vi "ArmSim.vi"(11 "Motor Dmd":dbl) -> (1 "Velocity_RadsPerSec":dbl, 2 "ArmAngle_Rad":dbl)   [LabVIEW 2023]
uses:
  <vilib>/Rock Robotics/WPI/ThirdParty/JAS_Junk/TrajLib/Enum/DCMOTOR_TYPES_ENUM.ctl
  <vilib>/Rock Robotics/WPI/ThirdParty/JAS_Junk/TrajLib/BatterySim_CalculateLoadedBatteryVoltage.vi
  <vilib>/Rock Robotics/WPI/ThirdParty/JAS_Junk/TrajLib/Trajectory_Library.lvlib
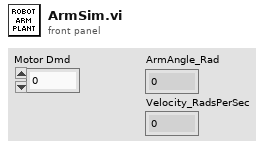
[diagram p1: front panel]
types:
  T1 = typedef "Trajectory_Library.lvlib/DCMOTOR_TYPES_ENUM.ctl" = enum16{"CIM", "AndyMark 9015", "Andy Mark RS 775 125", "Bag", "BaneBots RS 550", "BaneBots RS 775", "Falcon 500", "Mini CIM", "NEO", "NEO 550", "Romi BuiltIn", "Vex 775 Pro", "Snow Blower AM 2235A", "Bosch Seat AM 3493"}
  T2 = typedef "Trajectory_Library.lvlib/SINGLE_JOINT_ARM_SIM_SIMULATION_PARAMS.ctl" = cluster{"MinAngle_Rad":dbl, "MaxAngle_Rad":dbl, "Measurment StdDev":dbl, "SimulateGravity":bool}
  T3 = typedef "Trajectory_Library.lvlib/LINEAR_SYSTEM_ID_SINGLE_JOINT_ARM_MODEL.ctl" = cluster{"DCMOTOR_TYPES":T1, "Num Motors":i32, "ArmLength_M":dbl, "massKg":dbl, "Gearing":dbl, "MOI kgm2":dbl, "Estimate MOI":bool}
  T4 = typedef "Trajectory_Library.lvlib/SINGLE_JOINT_ARM_SIM.ctl" = cluster{"Arm_LinearSystem":T5, "GearBox":T8, "Gearing":dbl, "R_ArmLength_M":dbl, "MinAngle_Rad":dbl, "MaxAngle_Rad":dbl, "SimulateGravity":bool}
  T5 = typedef "Trajectory_Library.lvlib/LINEAR_SYSTEM_SIM.ctl" = cluster{"m_Plant":T6, "m_X":T7, "m_Y":T7, "m_U":T7, "MeasureStdDev":T7}
  T6 = typedef "Trajectory_Library.lvlib/LINEAR_SYSTEM.ctl" = cluster{"m_A":T7, "m_B":T7, "m_C":T7, "m_D":T7, "States":i32, "Inputs":i32, "Outputs":i32}
  T7 = typedef "NI_Matrix.lvlib/RealMatrix.ctl" = dbl[][]
  T8 = typedef "Trajectory_Library.lvlib/DCMOTOR.CTL" = cluster{"nominalVoltage_Volts":dbl, "StallTorque_NM":dbl, "StallCurrent_Amps":dbl, "FreeCurrent_Amps":dbl, "FreeSpeed_RadPerSec":dbl, "R_Ohms":dbl, "KvINV_RadPerSecPerVolt":dbl, "Kt_NMPerAmp":dbl, "L_H":dbl, "Jr_KgM2":dbl}
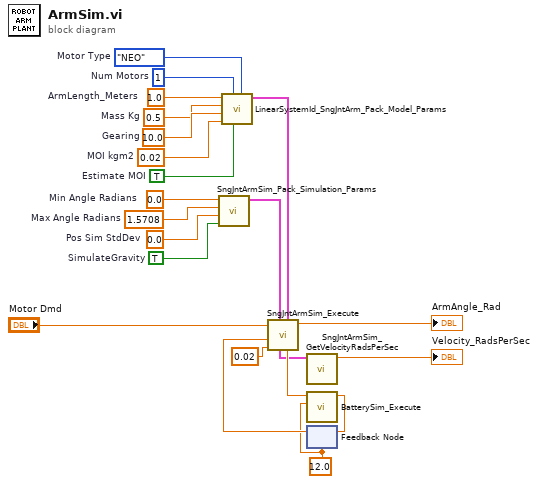
[diagram p0: block diagram]
diagram:
  w20 = 12.0 ("Battery Volts")
  w14 = TRUE  # Estimate MOI
  w13 = 0.02  # MOI kgm2
  w12 = 0.0  # Min Angle Radians
  w11 = 1.5708  # Max Angle Radians
  w10 = 0.0  # Pos Sim StdDev
  w9 = TRUE  # SimulateGravity
  w8 = 1.0  # ArmLength_Meters
  w7 = 10.0  # Gearing
  w6 = 0.5  # Mass Kg
  w5 = 1  # Num Motors
  w4 = DCMOTOR_TYPES_ENUM."NEO"  # Motor Type
  n1 = call <vilib>:"SngJntArmSim_Pack_Simulation_Params.vi"("SimulateGravity"=w9, "Pos Sim StdDev Rad"=w10, "MaxAngle_Rad"=w11, "MinAngle_Rad"=w12) -> ("SngJntArmSim_Simulation _Params"=w15:T2)  [unwired: 7 in]
  n2 = call <vilib>:"LinearSystemId_SngJntArm_Pack_Model_Params.vi"("DCMOTOR_TYPES"=w4, "Estimate MOI"=w14, "Num Motors"=w5, "MOI kgm2"=w13, "Gearing"=w7, "massKg"=w6, "ArmLength_M"=w8) -> ("SngJntArmSim_Model _Params"=w16:T3)  [unwired: 4 in]
  n3 = feedback #1(w20) -> (w22:dbl)
  n4 = call <vilib>:"SngJntArmSim_Execute.vi"("SngJntArmSim_Model _Params"=w16, "SngJntArmSim_Simulation _Params"=w15, "dT_Seconds"=0.02, "Battery Volts"=w22, "Motor Dmd"="Motor Dmd") -> ("ArmAngle_Rad"=→"ArmAngle_Rad":dbl, "Motor Current"=w21:dbl, "SingleJointArmSim"=w18:T4)  [unwired: 1 in, 3 out]
  n5 = call <vilib>:"SngJntArmSim_GetVelocityRadsPerSec.vi"("singleJointArmSim"=w18) -> ("Velocity_RadsPerSec"=→"Velocity_RadsPerSec":dbl)  [unwired: 10 in]
  n6 = call <vilib>:"BatterySim_Execute.vi"("Nominal Battery Voltage"=w20, "Current"=w21) -> ("Voltage"=w19:dbl)  [unwired: 9 in]
  n7 = feedback-in #1(w19) -> ()
